vi "Model 3566-Initialize.vi"(8 "error in":errorcluster, 11 "Model 3566 Setting In":T1) -> (0 "error out":errorcluster, 3 "Model 3566 Setting Out":T1)   [LabVIEW 2018]
uses:
  Data Def/Model 3566-Setting.ctl
  <vilib>/Instr/_visa.llb/VISA Configure Serial Port (Instr).vi
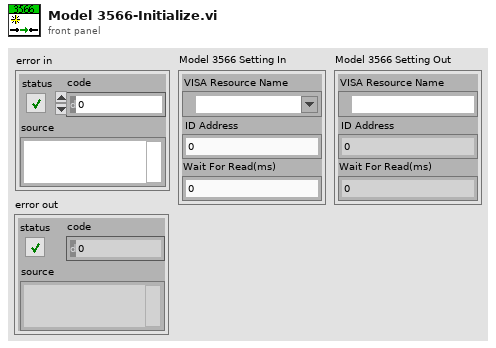
[diagram p1: front panel]
types:
  T1 = typedef "Model 3566-Setting.ctl" = cluster{"VISA Resource Name":refnum<visa-resource-name>, "ID Address":u8, "Wait For Read(ms)":u32}
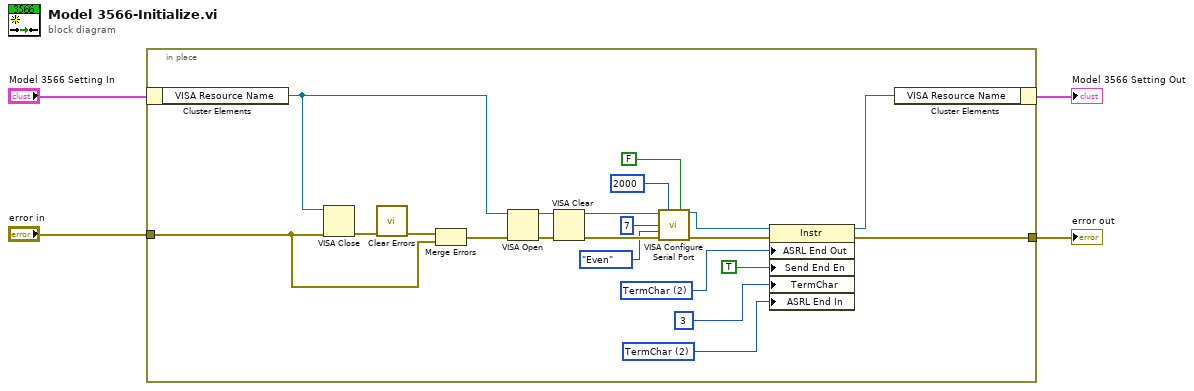
[diagram p0: block diagram]
diagram:
  n1 = in-place {
    in-place-border: "error in" -> [w10]
    in-place-border: [w11] -> w2
    w14 = u16 2 items=["None", "Last Bit", "TermChar", "Break"] ("Serial Settings:End Mode for Writes")
    w17 = u16 2 items=["None", "Last Bit", "TermChar", "Break"] ("Serial Settings:End Mode for Writes")
    n2 = in-place-cluster #1("Model 3566 Setting In") -> ("VISA Resource Name"=w12:refnum<visa-resource-name>)
    n3 = VISA Close(VISA resource name=w12, error in (no error)=w10) -> (error out=w25:errorcluster)
    n4 = call <vilib>:"Clear Errors.vi"("error in (no error)"=w25) -> ("error out"=w24:errorcluster)  [unwired: 5 in, 1 out]
    n5 = Merge Errors(w24, w10) -> (w13:errorcluster)
    n6 = VISA Open(error in (no error)=w13, VISA resource name=w12) -> (VISA resource name=w22:refnum<visa-resource-name>, error out=w23:errorcluster)  [unwired: 3 in]
    n7 = VISA Clear(VISA resource name=w22, error in (no error)=w23) -> (VISA resource name out=w20:refnum<visa-resource-name>, error out=w21:errorcluster)
    n8 = call-poly "VISA Configure Serial Port"("VISA resource name"=w20, "timeout (10sec)"=u32 2000, "Enable Termination\nChar (T)"=FALSE ("Enable Termination\nChar (T)"), "data bits (8)"=u16 7, "parity (0:none)"=enum16{"None", "Odd", "Even", "Mark", "Space"}."Even", "error in (no error)"=w21) -> ("VISA resource name out"=w18:refnum<visa-resource-name>, "error out"=w19:errorcluster)  [unwired: 8 in]
    n9 = property class="Instr"(reference=w18, error in=w19, "ASRL End Out"=w17, "Send End En"=TRUE ("Message Based Settings:Send End Enable"), "TermChar"=u8 3 ("Message Based Settings:Termination Character"), "ASRL End In"=w14) -> (reference out=w9:refnum<visa-resource-name>, error out=w11:errorcluster)
    n10 = in-place-cluster #1("VISA Resource Name"=w9) -> (→"Model 3566 Setting Out":T1)
  }
  "error out" <- w2
